vi "xlsx to Cluster (AIM - 1553).vi"(8 "Error (in)":errorcluster, 11 "file path (dialog if empty)":path) -> (0 "Error (out)":errorcluster, 2 "Parameter Array":T2[](array[typedef]), 3 "hw configuration":T1[](array[typedef])=[{"terminalAddress"=[3, 1, 0]}, {"terminalAddress"=[1, 0]}])   [LabVIEW 2020]
uses:
  _controls/aim1553_cluster.ctl
  _controls/aim1553_messages.ctl
  _controls/1553_Parameters_key.ctl
  _controls/1553_Parameters.ctl
  _controls/1553_minorFrames.ctl
  _controls/aim1553_RT_list.ctl
panel:
  out "data":string[][](array[string])
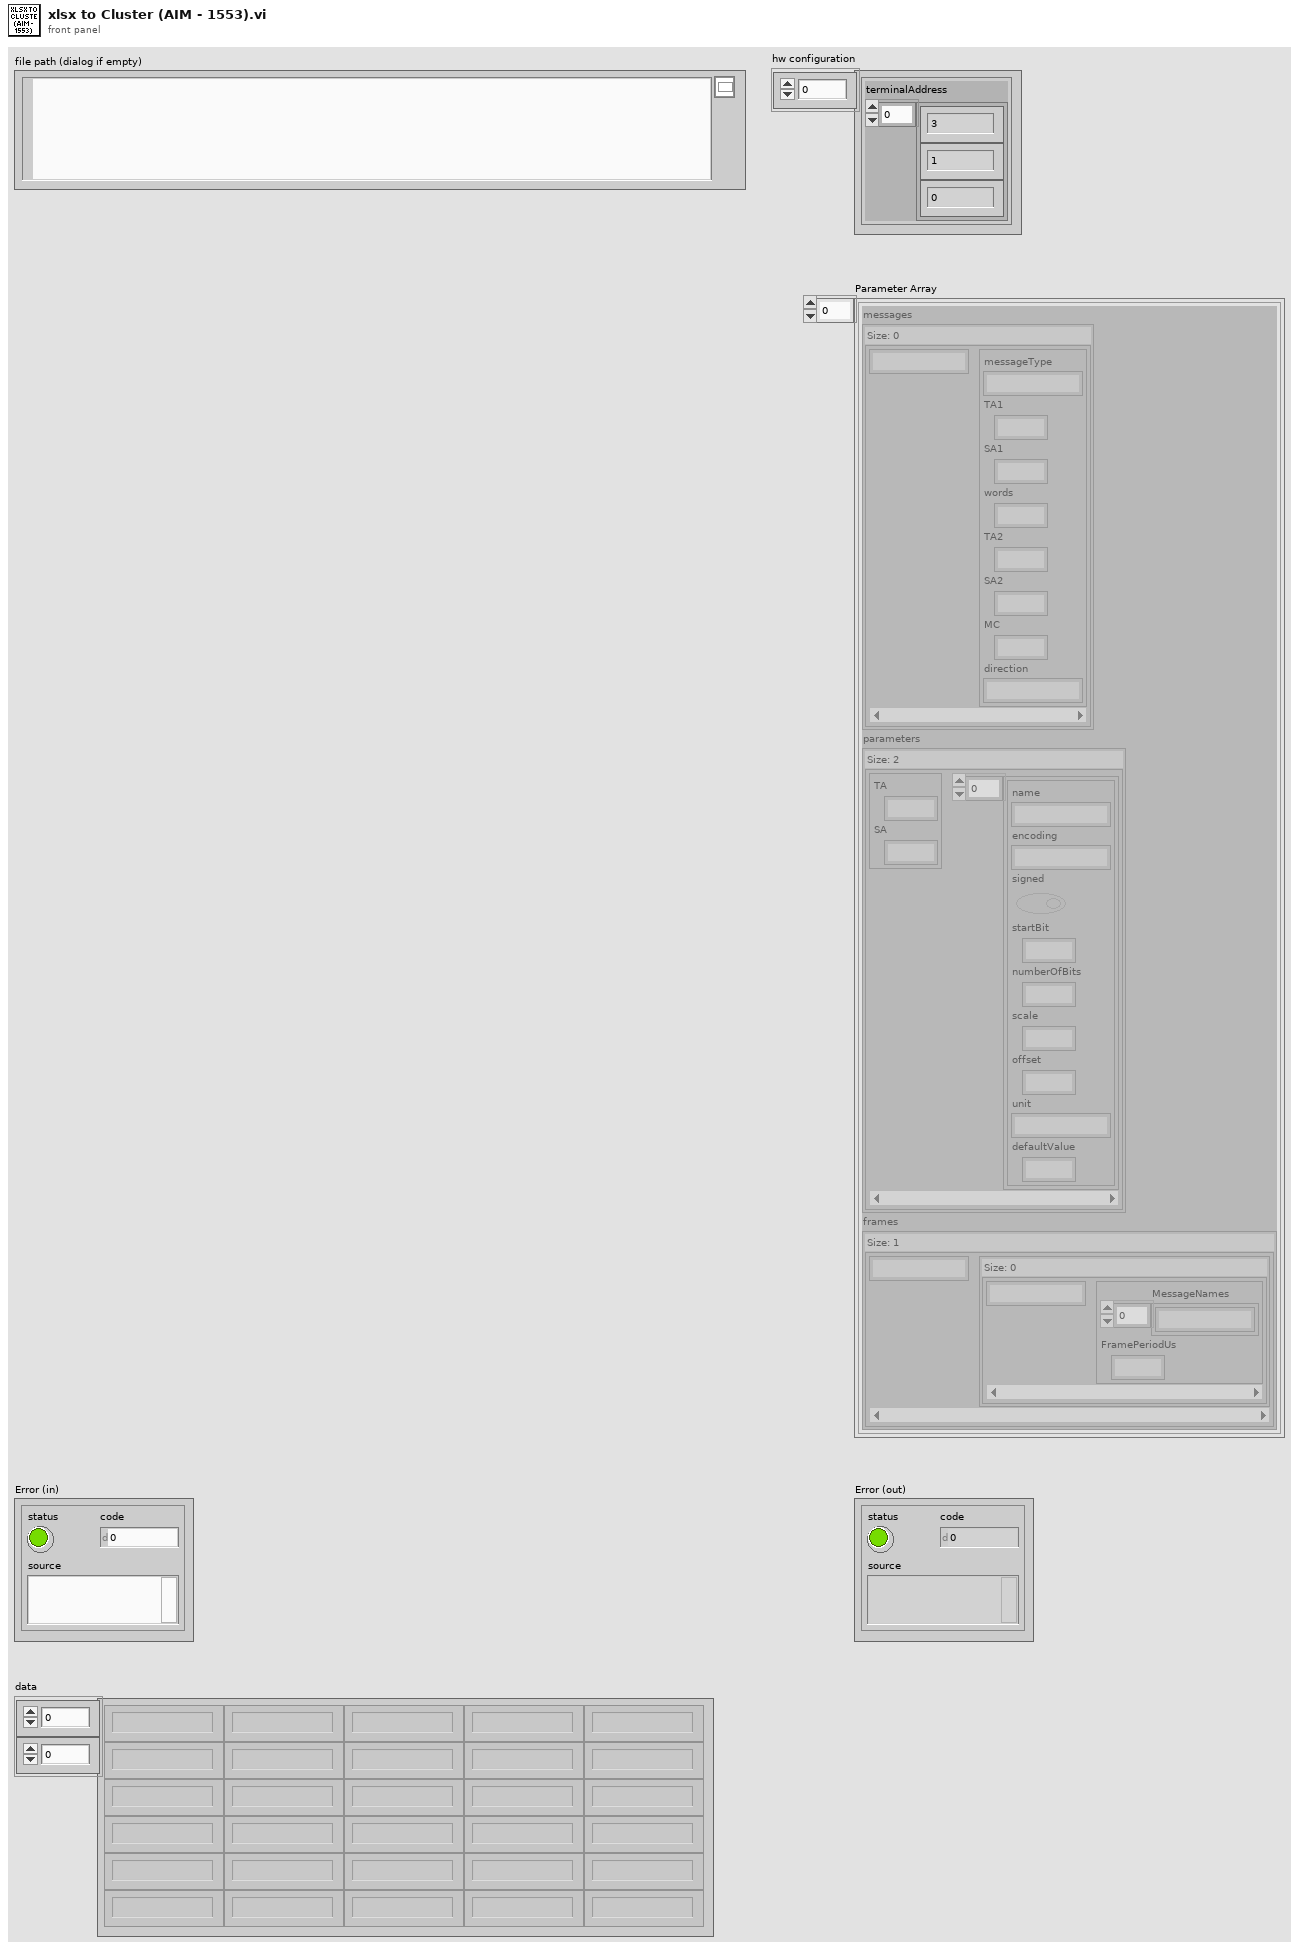
[diagram p1: front panel]
types:
  T1 = typedef "aim1553_RT_list.ctl" = cluster{"terminalAddress":i32[]}
  T2 = typedef "aim1553_cluster.ctl" = cluster{"messages":map{string, T3}, "parameters":map{T4, T5[]}, "frames":map{string, map{string, T6}}}
  T3 = typedef "aim1553_messages.ctl" = cluster{"messageType":string, "TA1":i32, "SA1":i32, "words":i32, "TA2":i32, "SA2":i32, "MC":i32, "direction":string}
  T4 = typedef "1553_Parameters_key.ctl" = cluster{"TA":i32, "SA":i32}
  T5 = typedef "1553_Parameters.ctl" = cluster{"name":string, "encoding":string, "signed":bool, "startBit":i32, "numberOfBits":i32, "scale":dbl, "offset":dbl, "unit":string, "defaultValue":dbl}
  T6 = typedef "1553_minorFrames.ctl" = cluster{"MessageNames":string[], "FramePeriodUs":i32}
  T7 = typedef "excelRefContainer.ctl" = cluster{"Application":refnum<k7>, "Workbooks":refnum<k7>, "Workbook":refnum<k7>}
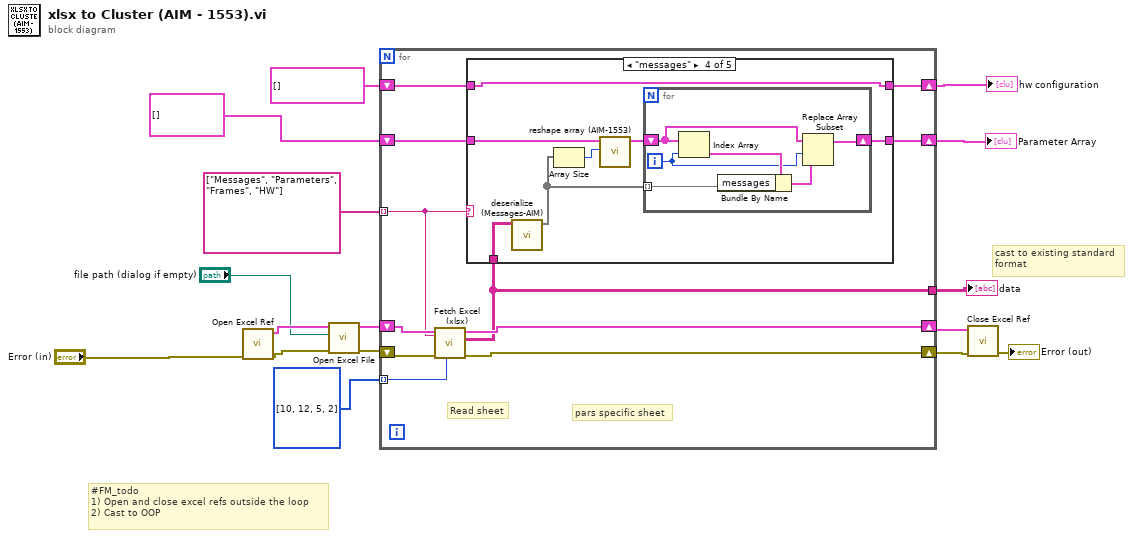
[diagram p0: block diagram]
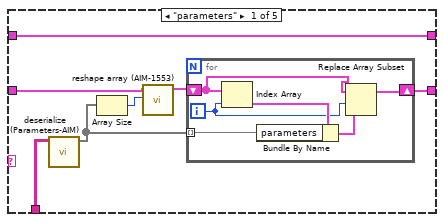
[diagram p2: hidden frame]
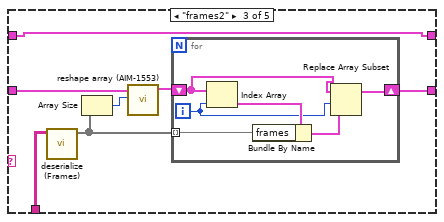
[diagram p4: hidden frame]
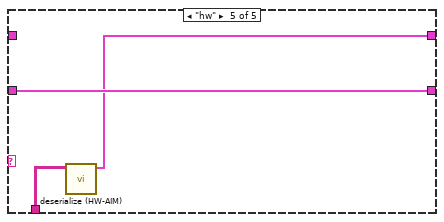
[diagram p5: hidden frame]
diagram:
  # "#FM_todo\n1) Open and close excel refs outside the loop\n2) Cast to OOP"
  # "cast to existing standard\nformat"
  n1 = call "Open Excel Ref.vi"("error in"="Error (in)") -> ("error out"=w12:errorcluster, "excelRefs out"=w11:T7)  [unwired: 9 in]
  n2 = call "Open Excel File.vi"("error in"=w12, "file path"="file path (dialog if empty)", "excelRefs in"=w11) -> ("error out"=w8:errorcluster, "excelRefs out"=w7:T7)  [unwired: 7 in]
  n3 = for {
    shift-right: [w25] -> w13
    shift-left: w8 -> [w24]
    tunnel: string[] ["Messages", "Parameters", "Frames", "HW"] -> [w22] mode=indexing
    tunnel: [w21] -> w15
    tunnel: i32[] [10, 12, 5, 2] ("columns (21)") -> [w23] mode=indexing
    shift-right: [w26] -> w5
    shift-left: w7 -> [w27]
    shift-right: [w19] -> w4
    shift-left: T2[] [] -> [w20]
    shift-right: [w17] -> w1
    shift-left: T1[] [] ("hw configuration") -> [w18]
    # "pars specific sheet"
    # "Read sheet"
    n4 = call "Fetch Excel (xlsx).vi"("columns (21)"=w23, "Excel._SheetName"=w22, "error in (no error)"=w24, "excelRefs in"=w27) -> ("error out"=w25:errorcluster, "data"=w21:string[][], "excelRefs out"=w26:T7)  [unwired: 5 in]
    n5 = case shown="\"messages\"" w22 {
      tunnel: w21 -> [w34 _ w49 w62 w70]
      tunnel: w20 -> [w30 w41 w47 w58 w71]
      tunnel: [w29 w41 w48 w59 w71] -> w19
      tunnel: w18 -> [w28 w42 w43 w56 _]
      tunnel: [w28 w42 w43 w56 w69] -> w17
      frame "parameters" {
        n6 = call "deserialize (Parameters-AIM).vi"("data in"=w34) -> ("parameters out"=w31:map{T4, T5[]}[])  [unwired: 10 in]
        n7 = Array Size(array=w31) -> (size(s)=w32:i32)
        n8 = call "reshape array (AIM-1553).vi"("size requested"=w32, "Array in"=w30) -> ("Array out"=w33:T2[])  [unwired: 9 in]
        n9 = for {
          shift-right: [w35] -> w29
          shift-left: w33 -> [w38]
          tunnel: w31 -> [w39] mode=indexing
          i -> [w37]
          n10 = Index Array(array=w38, index=w37) -> (element=w40:T2)
          n11 = Bundle By Name(cluster=w40, "parameters"=w39) -> (w36:T2)
          n12 = Replace Array Subset(array=w38, new element=w36, index=w37) -> (w35:T2[])
        }
      }
      frame Default {
      }
      frame "frames2" {
        n13 = call "deserialize (Frames).vi"("data in"=w49) -> ("frames"=w45:map{string, map{string, T6}}[])  [unwired: 10 in]
        n14 = Array Size(array=w45) -> (size(s)=w44:i32)
        n15 = call "reshape array (AIM-1553).vi"("size requested"=w44, "Array in"=w47) -> ("Array out"=w46:T2[])  [unwired: 9 in]
        n16 = for {
          shift-right: [w50] -> w48
          shift-left: w46 -> [w53]
          tunnel: w45 -> [w54] mode=indexing
          i -> [w52]
          n17 = Index Array(array=w53, index=w52) -> (element=w55:T2)
          n18 = Bundle By Name(cluster=w55, "frames"=w54) -> (w51:T2)
          n19 = Replace Array Subset(array=w53, new element=w51, index=w52) -> (w50:T2[])
        }
      }
      frame "messages" {
        n20 = call "deserialize (Messages-AIM).vi"("data in"=w62) -> ("messages"=w57:map{string, T3}[])  [unwired: 10 in]
        n21 = Array Size(array=w57) -> (size(s)=w60:i32)
        n22 = call "reshape array (AIM-1553).vi"("size requested"=w60, "Array in"=w58) -> ("Array out"=w61:T2[])  [unwired: 9 in]
        n23 = for {
          shift-right: [w64] -> w59
          shift-left: w61 -> [w67]
          tunnel: w57 -> [w63] mode=indexing
          i -> [w66]
          n24 = Index Array(array=w67, index=w66) -> (element=w68:T2)
          n25 = Bundle By Name(cluster=w68, "messages"=w63) -> (w65:T2)
          n26 = Replace Array Subset(array=w67, new element=w65, index=w66) -> (w64:T2[])
        }
      }
      frame "hw" {
        n27 = call "deserialize (HW-AIM).vi"("data in"=w70) -> ("hw configuration"=w69:T1[])  [unwired: 10 in]
      }
    }
  }
  "data" <- w15
  "Parameter Array" <- w4
  "hw configuration" <- w1
  n28 = call "Close Excel Ref.vi"("error in"=w13, "excelRefs in"=w5) -> ("error out"=→"Error (out)":errorcluster)  [unwired: 9 in]
